vi "DIO and LED operating point.vi"() -> ()   [LabVIEW 2013]
uses:
  <vilib>/Utility/file.llb/Read From Spreadsheet File (DBL).vi
panel:
  in  "[esc]":bool
  in  "Vdd [V]":dbl=3.3000000000000003 step=0.1
  in  "Rlim [ohms]":dbl(slide) scale=0.1..10000.0
  in  "Rout [ohms]":dbl=65.0
  in  "V-I logfile":path
  out "V-I plot":cluster{"all rows":dbl[], "all rows":dbl[]}[](graph)
  # "DIO / LED Operating Point"
  # "Digital output:"
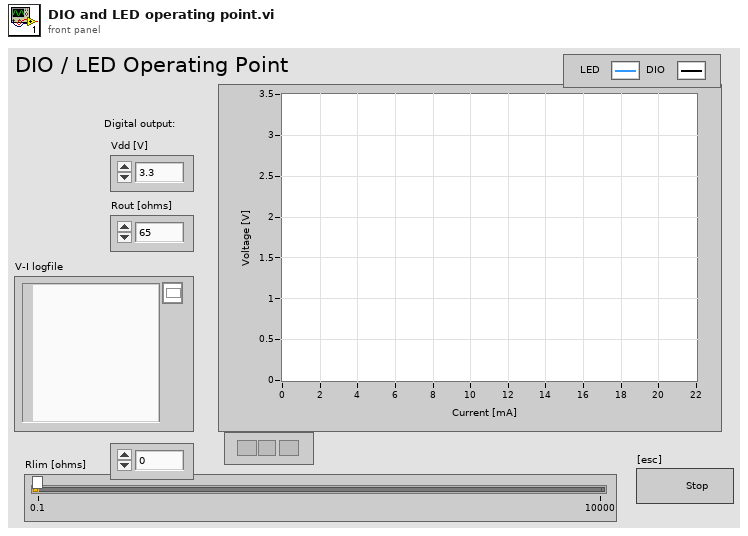
[diagram p1: front panel]
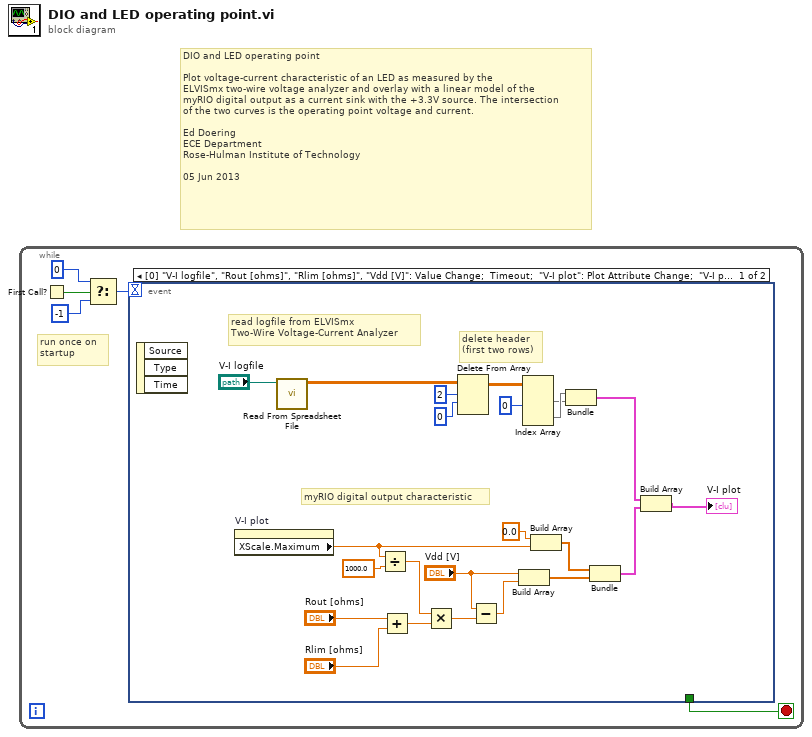
[diagram p0: block diagram]
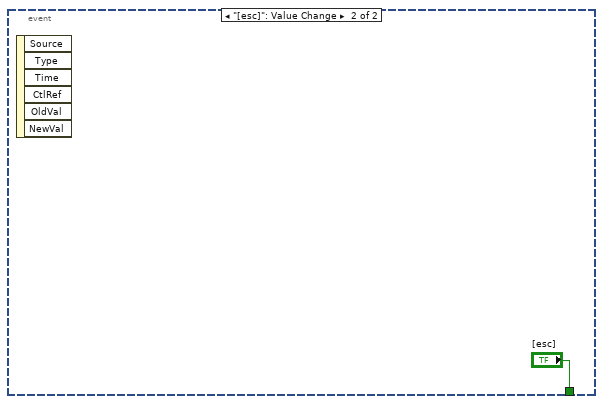
[diagram p2: hidden frame]
diagram:
  # "DIO and LED operating point\n\nPlot voltage-current characteristic of an LED as measured by the\nELVISmx two-wire voltage analyzer and overlay with a linear model of the\nmyRIO digital output as a current sink with the +3.3V source. The intersection\nof the two curves is the operating point voltage and current.\n\nEd Doering\nECE Department\nRose-Hulman Institute of Technology\n\n05 Jun 2013"
  n1 = while {
    stop <- w5 stop-if-true
    # "run once on \nstartup"
    n2 = First Call?() -> (First Call?: T/F=w2:bool)
    n3 = Select(t=0, s=w2, f=-1) -> (s? t:f=w4:i32)
    n4 = event shown="[0] \"V-I logfile\", \"Rout [ohms]\", \"Rlim [ohms]\", \"Vdd [V]\": Value Change;  Timeout;  \"V-I plot\": Plot Attribute Change;  \"V-I plot\": Autoscale Range Change;  \"V-I plot\": Scale Range Change" {
      selector: _ -> [_ _]
      dyn-events: _ -> [_ _]
      timeout: w4 -> [_ _]
      tunnel: [_ "[esc]"] -> w5
      event "V-I logfile", "Rout [ohms]", "Rlim [ohms]", "Vdd [V]": Value Change; Timeout; "V-I plot": Plot Attribute Change; "V-I plot": Autoscale Range Change; "V-I plot": Scale Range Change {
        # "myRIO digital output characteristic"
        # "read logfile from ELVISmx\nTwo-Wire Voltage-Current Analyzer"
        # "delete header\n(first two rows)"
        n5 = event-data() -> ()  [unwired: 1 in, 3 out]
        n6 = property on="V-I plot" class="XYGraph (strict)"() -> ("XScale.Maximum"=w13:dbl)  [unwired: 2 in, 2 out]
        n7 = call-poly <vilib>:"Read From Spreadsheet File.vi"("file path (dialog if empty)"="V-I logfile") -> ("all rows"=w28:dbl[][])  [unwired: 6 in, 4 out]
        n8 = Divide(x=w13, y=1000.0) -> (x/y=w14:dbl)
        n9 = Add(x="Rout [ohms]", y="Rlim [ohms]") -> (x+y=w17:dbl)
        n10 = Multiply(x=w14, y=w17) -> (x*y=w16:dbl)
        n11 = Delete From Array(array=w28, length=2, index (row)=0) -> (array with subset deleted=w25:dbl[][])  [unwired: 1 in, 1 out]
        n12 = Subtract(x="Vdd [V]", y=w16) -> (x-y=w6:dbl)
        n13 = Build Array("Vdd [V]", w6) -> (w8:dbl[])
        n14 = Index Array(array=w25, index (col) #1=0 ("disabled index (col)")) -> (element #1=w22:dbl[], element #2=w23:dbl[])  [unwired: 3 in]
        n15 = Build Array(0.0 ("element"), w13) -> (w10:dbl[])
        n16 = Bundle("all rows"=w23, "all rows"=w22) -> (w12:cluster{"all rows":dbl[], "all rows":dbl[]})  [unwired: 1 in]
        n17 = Bundle(w10, w8) -> (w9:cluster{dbl[], dbl[]})  [unwired: 1 in]
        n18 = Build Array(w12, w9) -> (→"V-I plot":cluster{"all rows":dbl[], "all rows":dbl[]}[])
      }
      event "[esc]": Value Change {
        n19 = event-data() -> ()  [unwired: 1 in, 6 out]
      }
    }
  }
